vi "002 Serial Port.vi"(11 "Queue Ref In":T1={"UI"=refnum, "Message"=refnum, "Data"=refnum, "Caller"=refnum, "Name"="000 Common", "Data Path"=path "", "Class Path"=path "", "SubPanel"=refnum, "Project Name"="", "MNT"="", "Title"="", "Data Source"=refnum, "Queue List"={}, "VI"=refnum, "UE"=refnum}) -> ()   [LabVIEW 2020]
doc: "Alin串口调试助手"
uses:
  Alin/QMH/000 Module Data Type.ctl
  Alin/QMH/Queue Message.ctl
panel:
  in  "Module Launch":bool
  in  "Delete":bool
  in  "Title":string="Alin串口调试助手"
  in  "Max":bool
  out "OPen":bool
  in  "数值":dbl
  in  "重复发送":bool
  in  "发送设置":enum32{"ASCII", "Hex"}(radio)
  in  "显示时间":bool
  in  "显示发送":bool
  in  "自动换行":bool
  in  "接收设置":enum32{"ASCII", "Hex"}(radio)
  in  "流控":u16(ring) items=["None", "RTS/CTS", "XON/XOFF"]
  in  "停止位":u16(ring) items=["1", "1.5", "2"]
  in  "校验位":u16(ring) items=["None", "Even", "Odd", "Mark", "Space"]
  in  "数据位":u16(ring)=3 items=["5", "6", "7", "8"]
  in  "BaudRate":u16(ring)=3 caption="波特率" items=["1200", "2400", "4800", "9600", "19200", "38400", "57600", "115200"]
  in  "Visa":refnum<visa-resource-name> caption="串口"
  in  "字符串 2":string
  in  "字符串":string
  in  "Send":bool
  in  "Tips":string="Welcome to use Alin Serial Port!"
  in  "Rx:":dbl format="%d Bytes"
  in  "Tx:":dbl format="%d Bytes"
  out "Time":string
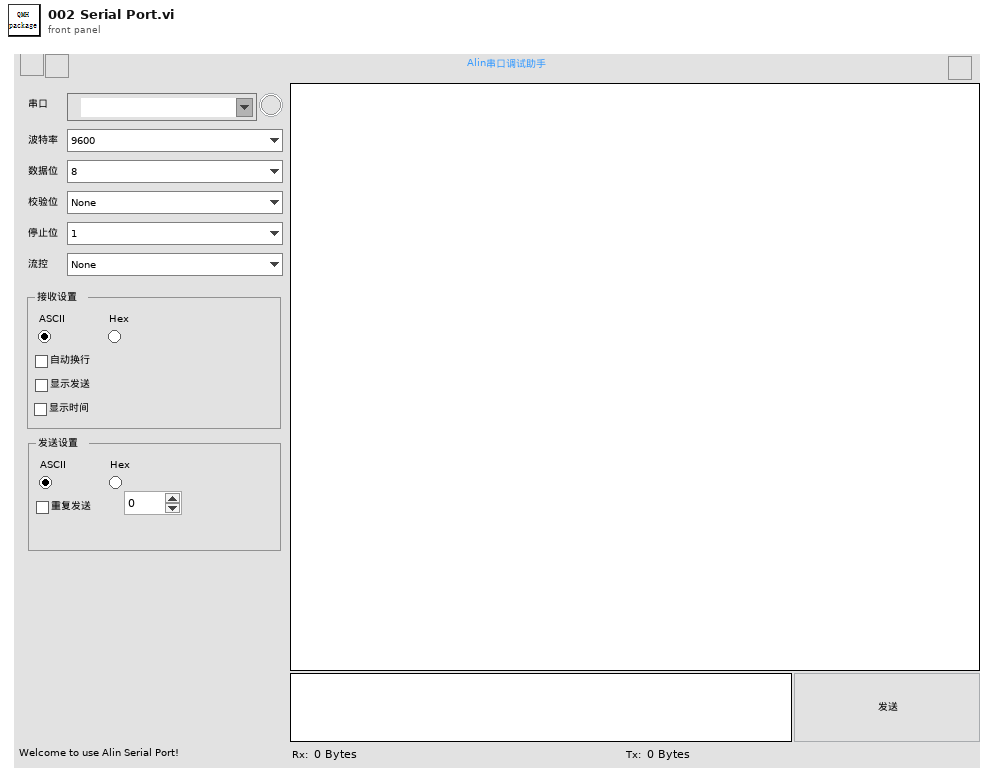
[diagram p1: front panel]
types:
  T1 = typedef "000 Module Data Type.ctl" = cluster{"UI":refnum<queue>, "Message":refnum<queue>, "Data":refnum<queue>, "Caller":refnum<queue>, "Name":string, "Data Path":path, "Class Path":path, "SubPanel":refnum<vi>, "Project Name":string, "MNT":string, "Title":string, "Data Source":refnum<queue>, "Queue List":map{string, refnum<queue>}, "VI":refnum<vi>, "UE":refnum<user-event>}
  T2 = cluster{"Queue":T1, "Delay":cluster{"Count Time(ms)":u32, "Delay Time(ms)":u32, "Next":string}}
  T3 = typedef "eventvkey.ctl" = enum16{"ASCII", "Enter", "Return", "Shift", "Ctrl", "Alt", "Cmd", "Opt", "Caps", "NumLock", "Clear", "Break", "Up", "Down", "Left", "Right", "Insert", "Delete", "Home", "End", "PageUp", "PageDown", "Escape", "Help", "Pause", "ScrollLock", "F1", "F2", "F3", "F4", "F5", "F6", "F7", "F8", "F9", "F10", "F11", "F12", "F13", "F14", "F15", "F16", "F17", "F18", "F19", "F20", "F21", "F22", "F23", "F24", "Play", "VolumeUp", "VolumeDown", "Mute", "Two Byte Char"}
  T4 = cluster{"Shift":bool, "Ctrl":bool, "Alt":bool, "Cmd":bool, "Opt":bool}
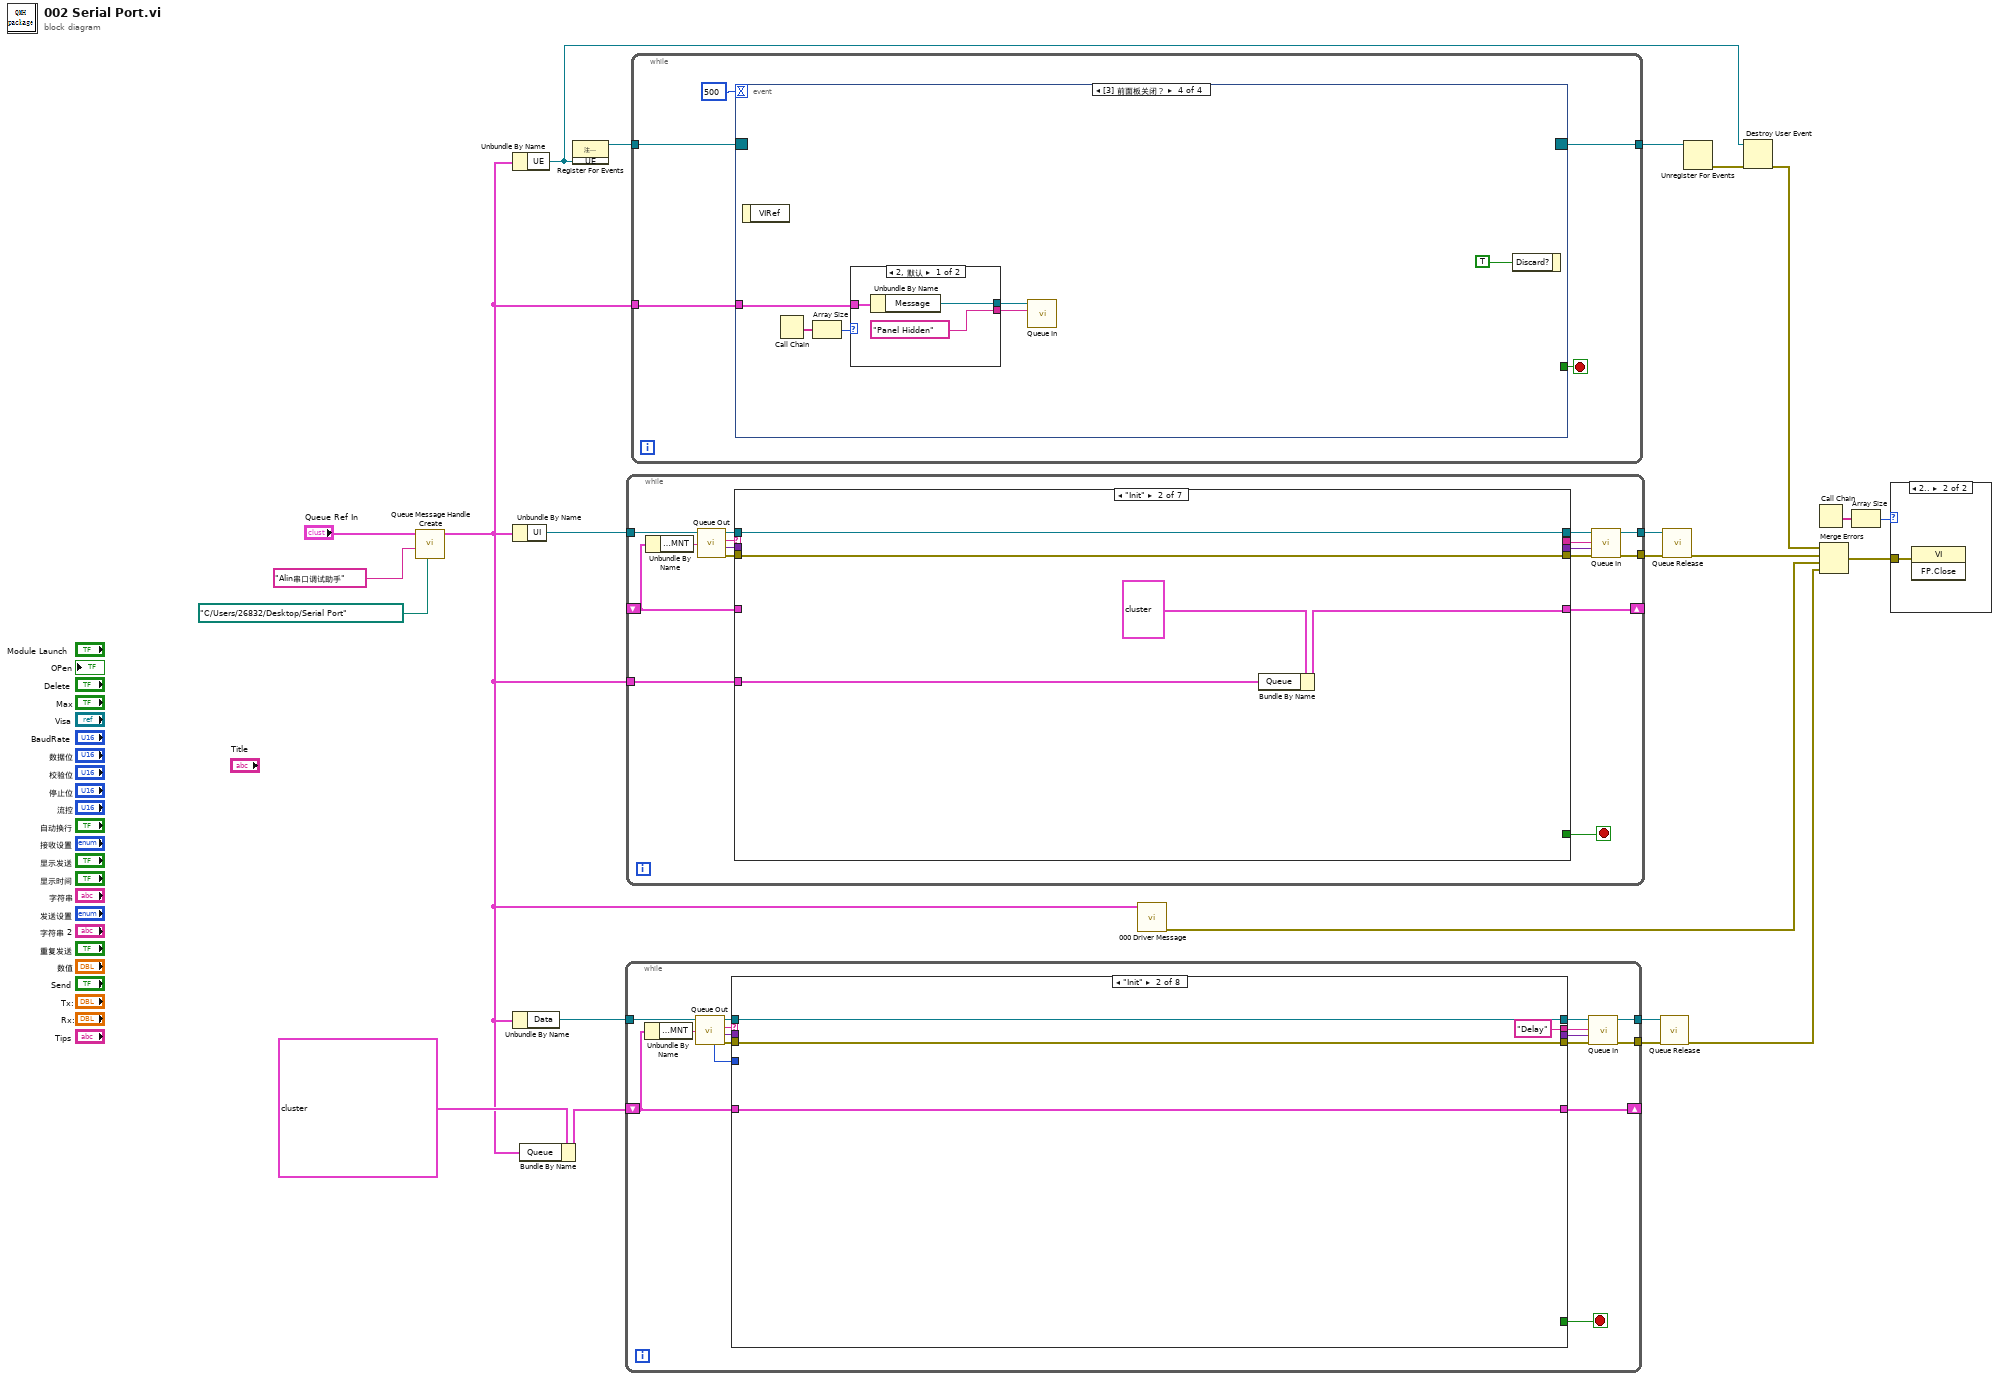
[diagram p0: block diagram]
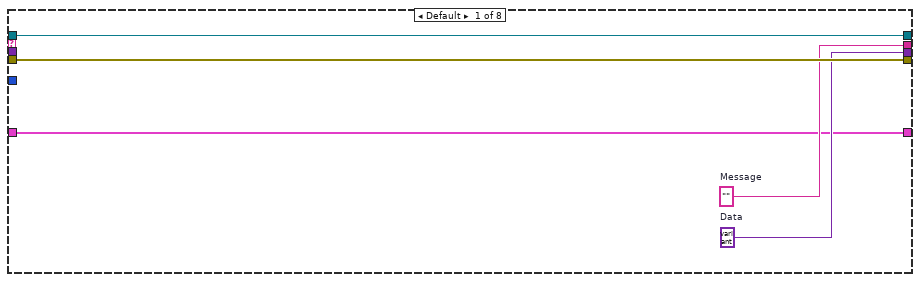
[diagram p2: hidden frame]
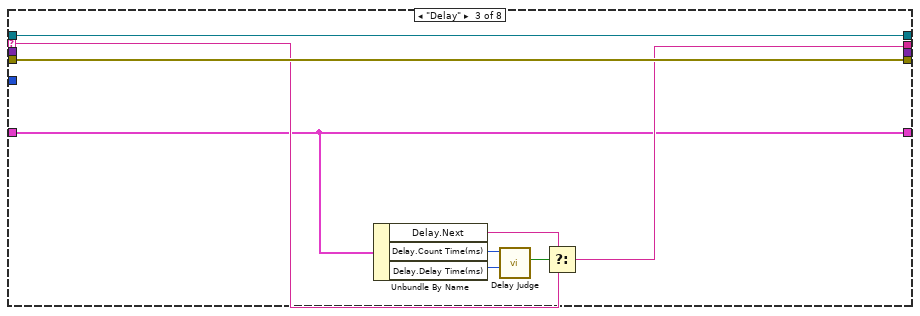
[diagram p3: hidden frame]
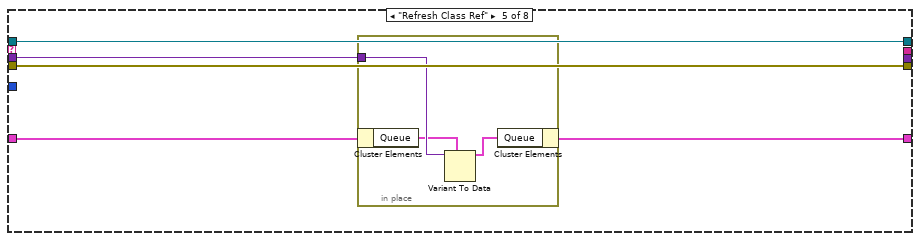
[diagram p5: hidden frame]
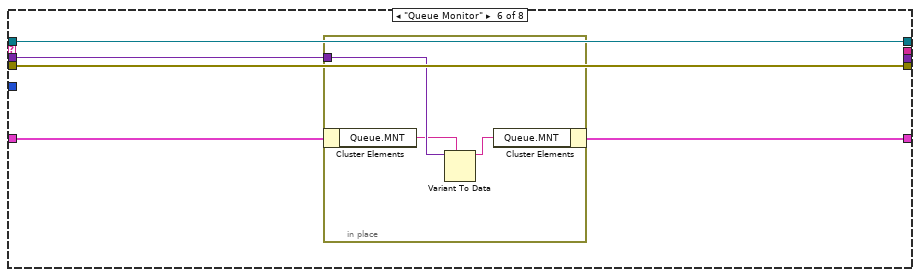
[diagram p6: hidden frame]
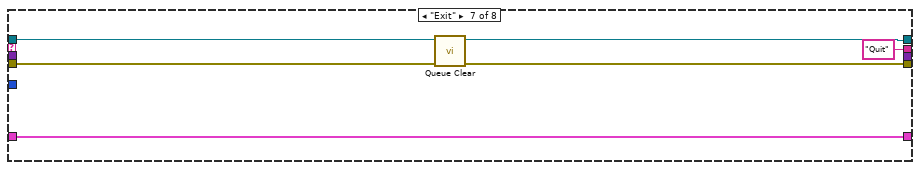
[diagram p7: hidden frame]
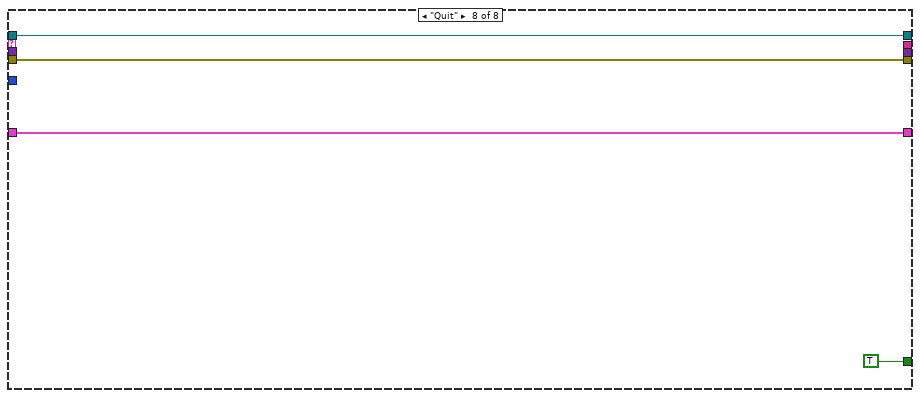
[diagram p8: hidden frame]
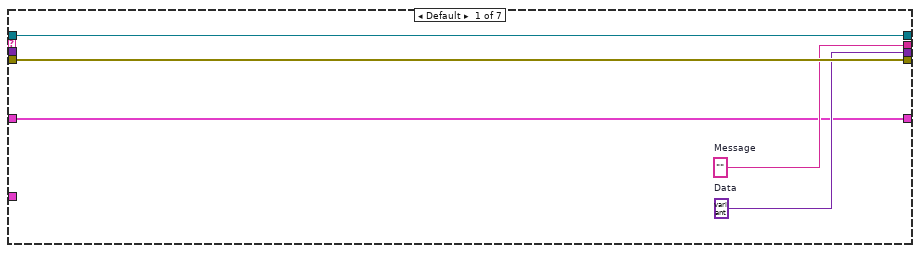
[diagram p10: hidden frame]
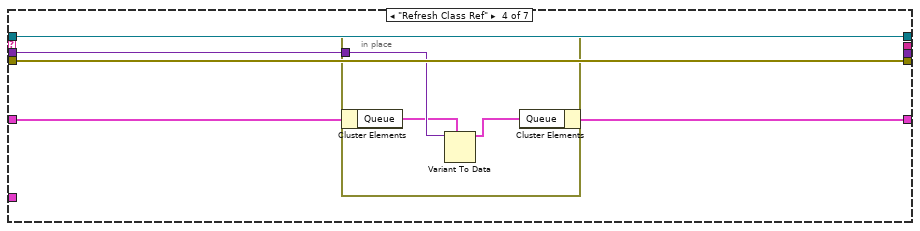
[diagram p12: hidden frame]
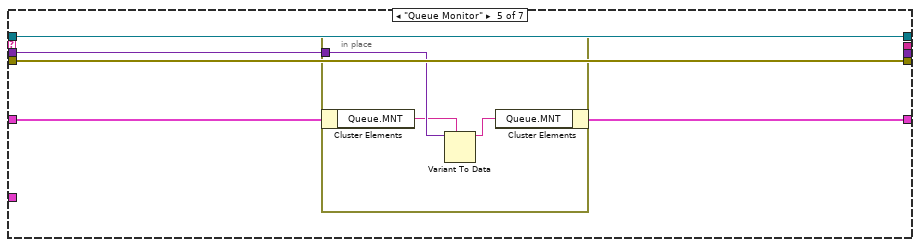
[diagram p13: hidden frame]
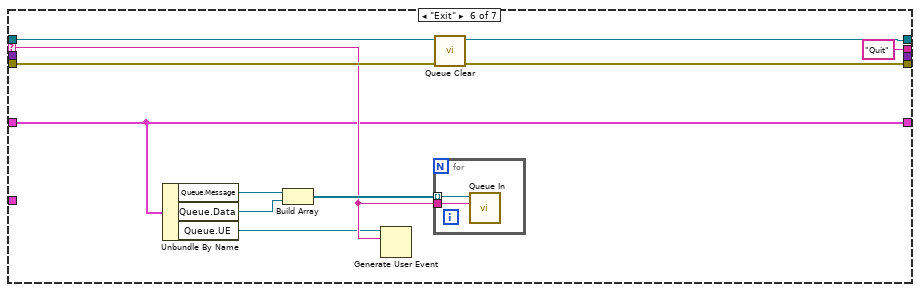
[diagram p14: hidden frame]
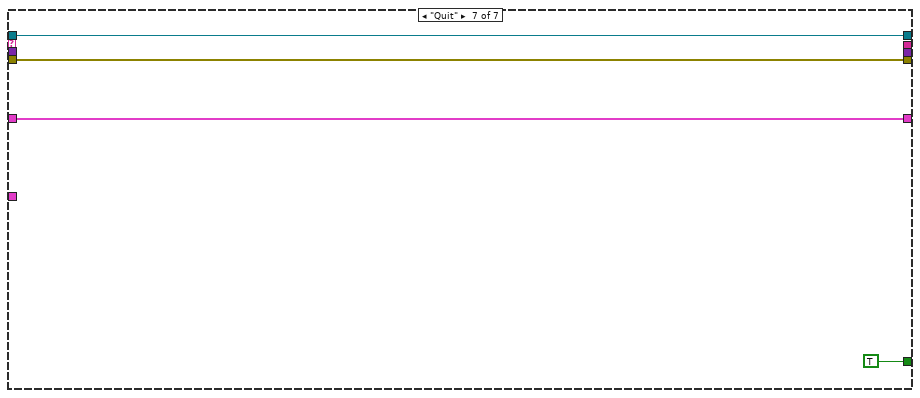
[diagram p15: hidden frame]
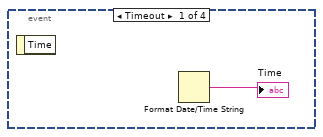
[diagram p16: hidden frame]
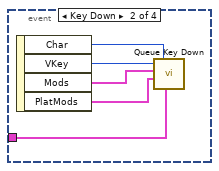
[diagram p17: hidden frame]
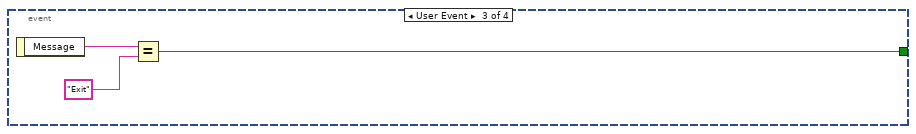
[diagram p18: hidden frame]
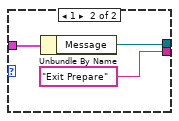
[diagram p19: hidden frame]
diagram:
  n1 = call "Queue Message Handle Create.vi"("Data Path"=path "C:/Users/26832/Desktop/Serial Port", "Name"="Alin串口调试助手", "Queue Ref In"="Queue Ref In") -> ("Queue Ref Out"=w2:T1)  [unwired: 7 in, 1 out]
  n2 = Unbundle By Name(w2) -> ("UE"=w7:refnum<user-event>)
  n3 = Unbundle By Name(w2) -> ("UI"=w18:refnum<queue>)
  n4 = Unbundle By Name(w2) -> ("Data"=w10:refnum<queue>)
  n5 = Bundle By Name(cluster=T2 {"Queue"={"UI"=refnum, "Message"=refnum, "Data"=refnum, "Caller"=refnum, "Name"="000 Common", "Data Path"=path "", "Class Path"=path "", "SubPanel"=refnum, "Project Name"="", "MNT"="", "Title"="", "Data Source"=refnum, "Queue List"={}, "VI"=refnum, "UE"=refnum}, "Delay"={"Count Time(ms)"=250, "Delay Time(ms)"=250, "Next"="Receive Data,Delay"}}, "Queue"=w2) -> (w3:T2)
  n6 = register-events(w7) -> (reference out=w23:refnum<event-registration>)  [unwired: 2 in, 1 out]
  n7 = while {
    tunnel: w10 -> [w35]
    tunnel: [w32] -> w12
    tunnel: [w31] -> w11
    shift-right: [w27] -> _
    shift-left: w3 -> [w24]
    stop <- w39 stop-if-true
    n8 = Unbundle By Name(w24) -> ("Queue.MNT"=w25:string)
    n9 = call "Queue Out.vi"("Monitor"=w25, "Queue In"=w35) -> ("error out"=w38:errorcluster, "Data"=w36:variant, "Message"=w37:string, "Queue Out"=w34:refnum<queue>, "Queue NUmber"=w26:i32)  [unwired: 5 in]
    n10 = case shown="\"Init\"" w37 {
      selector: w37 -> [_ _ w50 _ _ _ _ _]
      tunnel: w34 -> [w44 w48 w57 w60 w65 w73 w81 w85]
      tunnel: w38 -> [w43 w47 w56 w59 w64 w72 w79 w86]
      tunnel: [w44 w48 w57 w60 w65 w73 w80 w85] -> w33
      tunnel: [w43 w47 w56 w59 w64 w72 w78 w86] -> w30
      tunnel: [w42 "Delay" ("Next") w51 _ _ _ "Quit" _] -> w29
      tunnel: [_ _ _ _ _ _ _ TRUE] -> w39
      tunnel: [w41 _ _ _ _ _ _ _] -> w28
      tunnel: w36 -> [_ _ _ _ w61 w69 _ _]
      tunnel: [w40 w45 w49 w58 w62 w70 w77 w83] -> w27
      tunnel: w24 -> [w40 w45 w49 w58 w63 w71 w77 w83]
      tunnel: w26 -> [_ _ _ _ _ _ _ _]
      frame Default {
        w41 = variant  # Data
        w42 = ""  # Message
      }
      frame "Init" {
      }
      frame "Delay" {
        n11 = Unbundle By Name(w49) -> ("Delay.Next"=w55:string, "Delay.Count Time(ms)"=w52:u32, "Delay.Delay Time(ms)"=w53:u32)
        n12 = call "Delay Judge.vi"("Delay Time(ms)"=w53, "Count Time(ms)"=w52) -> ("Time Out?"=w54:bool)  [unwired: 5 in, 4 out]
        n13 = Select(t=w55, s=w54, f=w50) -> (s? t:f=w51:string)
      }
      frame "====System====" {
      }
      frame "Refresh Class Ref" {
        n14 = in-place {
          in-place-border: w61 -> [w68]
          n15 = in-place-cluster #1(w63) -> ("Queue"=w67:T1)
          n16 = Variant To Data(type=w67, Variant=w68) -> (data=w66:T1)  [unwired: 1 in, 1 out]
          n17 = in-place-cluster #1("Queue"=w66) -> (w62:T2)
        }
      }
      frame "Queue Monitor" {
        n18 = in-place {
          in-place-border: w69 -> [w76]
          n19 = in-place-cluster #2(w71) -> ("Queue.MNT"=w75:string)
          n20 = Variant To Data(type=w75, Variant=w76) -> (data=w74:string)  [unwired: 1 in, 1 out]
          n21 = in-place-cluster #2("Queue.MNT"=w74) -> (w70:T2)
        }
      }
      frame "Exit" {
        n22 = call "Queue Clear.vi"("error in (no error)"=w79, "Queue In"=w81) -> ("error out"=w78:errorcluster, "Queue Out"=w80:refnum<queue>)  [unwired: 8 in]
      }
      frame "Quit" {
      }
    }
    n23 = call "Queue In.vi"("error in (no error)"=w30, "Data"=w28, "Message"=w29, "Queue In"=w33) -> ("error out"=w31:errorcluster, "Queue Out"=w32:refnum<queue>)  [unwired: 6 in]
  }
  n24 = while {
    tunnel: w18 -> [w98]
    tunnel: [w95] -> w20
    tunnel: [w94] -> w19
    shift-right: [w90] -> _
    shift-left: _ -> [w89]
    tunnel: w2 -> [w87]
    stop <- w102 stop-if-true
    n25 = Unbundle By Name(w89) -> ("Queue.MNT"=w88:string)
    n26 = call "Queue Out.vi"("Monitor"=w88, "Queue In"=w98) -> ("error out"=w101:errorcluster, "Data"=w99:variant, "Message"=w100:string, "Queue Out"=w97:refnum<queue>)  [unwired: 5 in, 1 out]
    n27 = case shown="\"Init\"" w100 {
      selector: w100 -> [_ _ _ _ _ w134 _]
      tunnel: w97 -> [w107 w112 w115 w120 w128 w141 w147]
      tunnel: w101 -> [w106 w111 w114 w119 w127 w139 w148]
      tunnel: [w107 w112 w115 w120 w128 w140 w147] -> w96
      tunnel: [w106 w111 w114 w119 w127 w138 w148] -> w93
      tunnel: [w105 _ _ _ _ "Quit" _] -> w92
      tunnel: [_ _ _ _ _ _ TRUE] -> w102
      tunnel: [w104 _ _ _ _ _ _] -> w91
      tunnel: w99 -> [_ _ _ w116 w124 _ _]
      tunnel: [w103 w109 w113 w117 w125 w133 w145] -> w90
      tunnel: w89 -> [w103 _ w113 w118 w126 w133 w145]
      tunnel: w87 -> [_ w108 _ _ _ _ _]
      frame Default {
        w104 = variant  # Data
        w105 = ""  # Message
      }
      frame "Init" {
        n28 = Bundle By Name(cluster=cluster{"Queue":T1} {"Queue"={"UI"=refnum, "Message"=refnum, "Data"=refnum, "Caller"=refnum, "Name"="000 Common", "Data Path"=path "", "Class Path"=path "", "SubPanel"=refnum, "Project Name"="", "MNT"="", "Title"="", "Data Source"=refnum, "Queue List"={}, "VI"=refnum, "UE"=refnum}}, "Queue"=w108) -> (w109:cluster{"Queue":T1})
      }
      frame "====System====" {
      }
      frame "Refresh Class Ref" {
        n29 = in-place {
          in-place-border: w116 -> [w123]
          n30 = in-place-cluster #3(w118) -> ("Queue"=w122:T1)
          n31 = Variant To Data(type=w122, Variant=w123) -> (data=w121:T1)  [unwired: 1 in, 1 out]
          n32 = in-place-cluster #3("Queue"=w121) -> (w117:cluster{"Queue":T1})
        }
      }
      frame "Queue Monitor" {
        n33 = in-place {
          in-place-border: w124 -> [w131]
          n34 = in-place-cluster #4(w126) -> ("Queue.MNT"=w130:string)
          n35 = Variant To Data(type=w130, Variant=w131) -> (data=w129:string)  [unwired: 1 in, 1 out]
          n36 = in-place-cluster #4("Queue.MNT"=w129) -> (w125:cluster{"Queue":T1})
        }
      }
      frame "Exit" {
        n37 = Unbundle By Name(w133) -> ("Queue.Message"=w137:refnum<queue>, "Queue.Data"=w136:refnum<queue>, "Queue.UE"=w132:refnum<user-event>)
        n38 = Build Array(w137, w136) -> (w135:refnum<queue>[])
        n39 = Generate User Event(user event=w132, event data cluster=w134) -> ()  [unwired: 2 in, 2 out]
        n40 = for {
          tunnel: w135 -> [w144] mode=indexing
          tunnel: w134 -> [w143]
          n41 = call "Queue In.vi"("Message"=w143, "Queue In"=w144) -> ()  [unwired: 8 in, 2 out]
        }
        n42 = call "Queue Clear.vi"("error in (no error)"=w139, "Queue In"=w141) -> ("error out"=w138:errorcluster, "Queue Out"=w140:refnum<queue>)  [unwired: 8 in]
      }
      frame "Quit" {
      }
    }
    n43 = call "Queue In.vi"("error in (no error)"=w93, "Data"=w91, "Message"=w92, "Queue In"=w96) -> ("error out"=w94:errorcluster, "Queue Out"=w95:refnum<queue>)  [unwired: 6 in]
  }
  n44 = while {
    tunnel: w23 -> [w153]
    tunnel: [w151] -> w22
    tunnel: w2 -> [w150]
    stop <- w152 stop-if-true
    n45 = event shown="[3] 前面板关闭？" {
      selector: w153 -> [_ _ _ _]
      dyn-events: [_ _ _ _] -> w151
      timeout: 500 -> [_ _ _ _]
      tunnel: [_ _ w160 _] -> w152
      tunnel: w150 -> [_ w158 _ w165]
      event Timeout {
        n46 = event-data() -> ()  [unwired: 1 in, 1 out]
        n47 = Format Date/Time String() -> (date/time string=→"Time":string)  [unwired: 3 in]
      }
      event Key Down {
        n48 = event-data() -> ("Char"=w159:i16, "VKey"=w157:T3, "Mods"=w156:cluster{"Num Pad":bool, "Menu Key":bool}, "PlatMods"=w155:T4)  [unwired: 1 in]
        n49 = call "Queue Key Down.vi"("Queue Ref Out"=w158, "C"=w159, "Platform Key"=w155, "Group Key"=w156, "V Key"=w157) -> ()  [unwired: 6 in, 1 out]
      }
      event User Event {
        n50 = event-data() -> ("Message"=w162:string)  [unwired: 1 in]
        n51 = Equal?(x=w162, y="Exit") -> (x = y?=w160:bool)
      }
      event Panel Close? {
        n52 = event-data() -> ()  [unwired: 1 in, 1 out]
        n53 = Call Chain() -> (call chain=w167:string[])
        n54 = Array Size(array=w167) -> (size(s)=w166:i32)
        n55 = case shown="2, 默认" w166 {
          tunnel: w165 -> [w171 w174]
          tunnel: [w170 w173] -> w164
          tunnel: ["Panel Hidden" ("Message") "Exit Prepare" ("Message")] -> w163
          frame 2, Default {
            n56 = Unbundle By Name(w171) -> ("Message"=w170:refnum<queue>)
          }
          frame 1 {
            n57 = Unbundle By Name(w174) -> ("Message"=w173:refnum<queue>)
          }
        }
        n58 = call "Queue In.vi"("Message"=w163, "Queue In"=w164) -> ()  [unwired: 8 in, 2 out]
        n59 = event-data("Discard?"=TRUE ("放弃？")) -> ()  [unwired: 1 in, 1 out]
      }
    }
  }
  n60 = call "000 Driver Message.vi"("Queue In"=w2) -> ("error out"=w8:errorcluster)  [unwired: 8 in, 2 out]
  n61 = call "Queue Release.vi"("error in (no error)"=w11, "Queue In"=w12) -> ("error out"=w9:errorcluster)  [unwired: 9 in]
  n62 = call "Queue Release.vi"("error in (no error)"=w19, "Queue In"=w20) -> ("error out"=w16:errorcluster)  [unwired: 9 in]
  n63 = Unregister For Events(event registration refnum=w22) -> (error out=w21:errorcluster)  [unwired: 1 in]
  n64 = Destroy User Event(user event=w7, error in=w21) -> (error out=w17:errorcluster)
  n65 = Call Chain() -> (call chain=w14:string[])
  n66 = Merge Errors(w17, w16, w8, w9) -> (w15:errorcluster)
  n67 = Array Size(array=w14) -> (size(s)=w13:i32)
  n68 = case shown="2.." w13 {
    tunnel: w15 -> [_ w175]
    frame 0, Default {
    }
    frame 2.. {
      n69 = invoke class="VI" method="FP.Close"(error in=w175) -> ()  [unwired: 2 in, 3 out]
    }
  }
